vi "Read Level.vi"(8 "error in (no error)":errorcluster, 11 "Logger in":refnum<class "Logger.lvclass">) -> (0 "error out":errorcluster, 2 "Level":T1, 3 "Logger out":refnum<class "Logger.lvclass">)   [LabVIEW 2022 SP3, in "Logger.lvlib" / "Logger.lvclass"]
uses:
  Logger.lvclass
  Logger.lvclass/Logger.ctl
  _Level.ctl
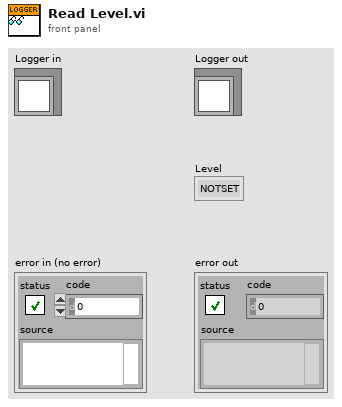
[diagram p1: front panel]
types:
  T1 = typedef "Logger.lvlib/Logger.lvclass/_Level.ctl" = enum16{"NOTSET", "DEBUG", "INFO", "WARNING", "ERROR", "CRITICAL"}
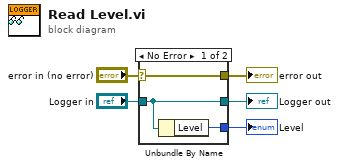
[diagram p0: block diagram]
diagram:
  n1 = case shown="No Error" "error in (no error)" {
    selector: "error in (no error)" -> [w8 w9]
    tunnel: [w8 w9] -> w4
    tunnel: [w7 w10] -> w2
    tunnel: "Logger in" -> [w7 w10]
    tunnel: [w6 _] -> w1
    frame No Error {
      n2 = Unbundle By Name(w7) -> ("Level"=w6:T1)
    }
    frame Error {
    }
  }
  "error out" <- w4
  "Logger out" <- w2
  "Level" <- w1
